vi "MJG_offsetEncCnts.vi"(8 "XYZ Offsets [enc cnts]":i32[](array[numeric]), 9 "Z Stage Enc Count":i32, 10 "Y Stage Enc Count":i32, 11 "X Stage Enc Count":i32) -> (1 "Z Stage [abs enc cnt]":i32, 2 "Y Stage [abs enc cnt]":i32, 3 "X Stage [abs enc cnt]":i32)   [LabVIEW 2016]
panel:
  # ">>>"
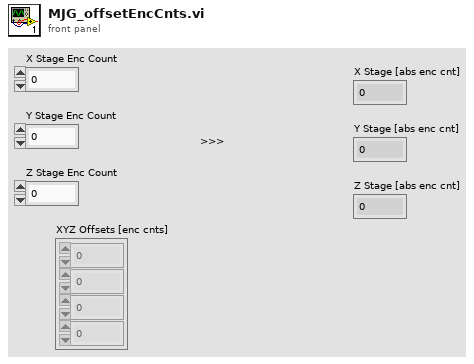
[diagram p1: front panel]
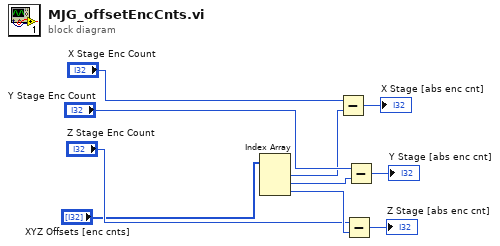
[diagram p0: block diagram]
diagram:
  n1 = Index Array(array="XYZ Offsets [enc cnts]") -> (element #1=w3:i32, element #2=w5:i32, element #3=w7:i32)  [unwired: 3 in]
  n2 = Subtract(x="X Stage Enc Count", y=w3) -> (x-y=→"X Stage [abs enc cnt]":i32)
  n3 = Subtract(x="Z Stage Enc Count", y=w7) -> (x-y=→"Z Stage [abs enc cnt]":i32)
  n4 = Subtract(x="Y Stage Enc Count", y=w5) -> (x-y=→"Y Stage [abs enc cnt]":i32)
